vi "Write Autonomous.vi"() -> ()   [LabVIEW 2011]
uses:
  Shared/Autonomous Recording TypeDef.ctl
panel:
  in  "Autonomous Array":T1[](array[typedef])=[{"Left Drive Encoder"=0.0, "Right Drive Encoder"=0.0, "Shooter Mode"=enum."Off", "Set RPM"=0.0, "Set Motor Speed"=0.0, "Horn"=FALSE, "Shift Low"=FALSE, "Shift High"=FALSE, "Fire"=FALSE, "Reset Encoders"=FALSE}, {"Left Drive Encoder"=0.0, "Right Drive Encoder"=0.0, "Shooter Mode"=enum."Off", "Set RPM"=0.0, "Set Motor Speed"=0.0, "Horn"=FALSE, "Shift Low"=FALSE, "Shift High"=FALSE, "Fire"=FALSE, "Reset Encoders"=FALSE}, {"Left Drive Encoder"=0.0, "Right Drive Encoder"=0.0, "Shooter Mode"=enum."Off", "Set RPM"=0.0, "Set Motor Speed"=0.0, "Horn"=FALSE, "Shift Low"=FALSE, "Shift High"=FALSE, "Fire"=FALSE, "Reset Encoders"=FALSE}, {"Left Drive Encoder"=0.0, "Right Drive Encoder"=0.0, "Shooter Mode"=enum."Off", "Set RPM"=0.0, "Set Motor Speed"=0.0, "Horn"=FALSE, "Shift Low"=FALSE, "Shift High"=FALSE, "Fire"=FALSE, "Reset Encoders"=FALSE}, {"Left Drive Encoder"=0.0, "Right Drive Encoder"=0.0, "Shooter Mode"=enum."Off", "Set RPM"=0.0, "Set Motor Speed"=0.0, "Horn"=FALSE, "Shift Low"=FALSE, "Shift High"=FALSE, "Fire"=FALSE, "Reset Encoders"=FALSE}, {"Left Drive Encoder"=0.0, "Right Drive Encoder"=0.0, "Shooter Mode"=enum."Off", "Set RPM"=0.0, "Set Motor Speed"=0.0, "Horn"=FALSE, "Shift Low"=FALSE, "Shift High"=FALSE, "Fire"=FALSE, "Reset Encoders"=FALSE}, {"Left Drive Encoder"=0.0, "Right Drive Encoder"=0.0, "Shooter Mode"=enum."Off", "Set RPM"=0.0, "Set Motor Speed"=0.0, "Horn"=FALSE, "Shift Low"=FALSE, "Shift High"=FALSE, "Fire"=FALSE, "Reset Encoders"=FALSE}, {"Left Drive Encoder"=0.0, "Right Drive Encoder"=0.0, "Shooter Mode"=enum."Off", "Set RPM"=0.0, "Set Motor Speed"=0.0, "Horn"=FALSE, "Shift Low"=FALSE, "Shift High"=FALSE, "Fire"=FALSE, "Reset Encoders"=FALSE}, {"Left Drive Encoder"=0.0, "Right Drive Encoder"=0.0, "Shooter Mode"=enum."Off", "Set RPM"=0.0, "Set Motor Speed"=0.0, "Horn"=FALSE, "Shift Low"=FALSE, "Shift High"=FALSE, "Fire"=FALSE, "Reset Encoders"=FALSE}, {"Left Drive Encoder"=0.0, "Right Drive Encoder"=0.0, "Shooter Mode"=enum."Off", "Set RPM"=0.0, "Set Motor Speed"=0.0, "Horn"=FALSE, "Shift Low"=FALSE, "Shift High"=FALSE, "Fire"=FALSE, "Reset Encoders"=FALSE}, {"Left Drive Encoder"=0.0, "Right Drive Encoder"=0.0, "Shooter Mode"=enum."Off", "Set RPM"=0.0, "Set Motor Speed"=0.0, "Horn"=FALSE, "Shift Low"=FALSE, "Shift High"=FALSE, "Fire"=FALSE, "Reset Encoders"=FALSE}, {"Left Drive Encoder"=0.0, "Right Drive Encoder"=0.0, "Shooter Mode"=enum."Off", "Set RPM"=0.0, "Set Motor Speed"=0.0, "Horn"=FALSE, "Shift Low"=FALSE, "Shift High"=FALSE, "Fire"=FALSE, "Reset Encoders"=FALSE}, {"Left Drive Encoder"=0.0, "Right Drive Encoder"=0.0, "Shooter Mode"=enum."Off", "Set RPM"=0.0, "Set Motor Speed"=0.0, "Horn"=FALSE, "Shift Low"=FALSE, "Shift High"=FALSE, "Fire"=FALSE, "Reset Encoders"=FALSE}, {"Left Drive Encoder"=0.0, "Right Drive Encoder"=0.0, "Shooter Mode"=enum."Off", "Set RPM"=0.0, "Set Motor Speed"=0.0, "Horn"=FALSE, "Shift Low"=FALSE, "Shift High"=FALSE, "Fire"=FALSE, "Reset Encoders"=FALSE}, {"Left Drive Encoder"=0.0, "Right Drive Encoder"=0.0, "Shooter Mode"=enum."Off", "Set RPM"=0.0, "Set Motor Speed"=0.0, "Horn"=FALSE, "Shift Low"=FALSE, "Shift High"=FALSE, "Fire"=FALSE, "Reset Encoders"=FALSE}, {"Left Drive Encoder"=0.0, "Right Drive Encoder"=0.0, "Shooter Mode"=enum."Off", "Set RPM"=0.0, "Set Motor Speed"=0.0, "Horn"=FALSE, "Shift Low"=FALSE, "Shift High"=FALSE, "Fire"=FALSE, "Reset Encoders"=FALSE}, {"Left Drive Encoder"=0.0, "Right Drive Encoder"=0.0, "Shooter Mode"=enum."Off", "Set RPM"=0.0, "Set Motor Speed"=0.0, "Horn"=FALSE, "Shift Low"=FALSE, "Shift High"=FALSE, "Fire"=FALSE, "Reset Encoders"=FALSE}, {"Left Drive Encoder"=0.0, "Right Drive Encoder"=0.0, "Shooter Mode"=enum."Off", "Set RPM"=0.0, "Set Motor Speed"=0.0, "Horn"=FALSE, "Shift Low"=FALSE, "Shift High"=FALSE, "Fire"=FALSE, "Reset Encoders"=FALSE}, {"Left Drive Encoder"=0.0, "Right Drive Encoder"=0.0, "Shooter Mode"=enum."Off", "Set RPM"=0.0, "Set Motor Speed"=0.0, "Horn"=FALSE, "Shift Low"=FALSE, "Shift High"=FALSE, "Fire"=FALSE, "Reset Encoders"=FALSE}, {"Left Drive Encoder"=0.0, "Right Drive Encoder"=0.0, "Shooter Mode"=enum."Off", "Set RPM"=0.0, "Set Motor Speed"=0.0, "Horn"=FALSE, "Shift Low"=FALSE, "Shift High"=FALSE, "Fire"=FALSE, "Reset Encoders"=FALSE}, {"Left Drive Encoder"=0.0, "Right Drive Encoder"=0.0, "Shooter Mode"=enum."Off", "Set RPM"=0.0, "Set Motor Speed"=0.0, "Horn"=FALSE, "Shift Low"=FALSE, "Shift High"=FALSE, "Fire"=FALSE, "Reset Encoders"=FALSE}, {"Left Drive Encoder"=0.0, "Right Drive Encoder"=0.0, "Shooter Mode"=enum."Off", "Set RPM"=0.0, "Set Motor Speed"=0.0, "Horn"=FALSE, "Shift Low"=FALSE, "Shift High"=FALSE, "Fire"=FALSE, "Reset Encoders"=FALSE}, {"Left Drive Encoder"=0.0, "Right Drive Encoder"=0.0, "Shooter Mode"=enum."Off", "Set RPM"=0.0, "Set Motor Speed"=0.0, "Horn"=FALSE, "Shift Low"=FALSE, "Shift High"=FALSE, "Fire"=FALSE, "Reset Encoders"=FALSE}, {"Left Drive Encoder"=0.0, "Right Drive Encoder"=0.0, "Shooter Mode"=enum."Off", "Set RPM"=0.0, "Set Motor Speed"=0.0, "Horn"=FALSE, "Shift Low"=FALSE, "Shift High"=FALSE, "Fire"=FALSE, "Reset Encoders"=FALSE}, {"Left Drive Encoder"=0.0, "Right Drive Encoder"=0.0, "Shooter Mode"=enum."Off", "Set RPM"=0.0, "Set Motor Speed"=0.0, "Horn"=FALSE, "Shift Low"=FALSE, "Shift High"=FALSE, "Fire"=FALSE, "Reset Encoders"=FALSE}, {"Left Drive Encoder"=0.0, "Right Drive Encoder"=0.0, "Shooter Mode"=enum."Off", "Set RPM"=0.0, "Set Motor Speed"=0.0, "Horn"=FALSE, "Shift Low"=FALSE, "Shift High"=FALSE, "Fire"=FALSE, "Reset Encoders"=FALSE}, {"Left Drive Encoder"=0.0, "Right Drive Encoder"=0.0, "Shooter Mode"=enum."Off", "Set RPM"=0.0, "Set Motor Speed"=0.0, "Horn"=FALSE, "Shift Low"=FALSE, "Shift High"=FALSE, "Fire"=FALSE, "Reset Encoders"=FALSE}, {"Left Drive Encoder"=0.0, "Right Drive Encoder"=0.0, "Shooter Mode"=enum."Off", "Set RPM"=0.0, "Set Motor Speed"=0.0, "Horn"=FALSE, "Shift Low"=FALSE, "Shift High"=FALSE, "Fire"=FALSE, "Reset Encoders"=FALSE}, {"Left Drive Encoder"=0.0, "Right Drive Encoder"=0.0, "Shooter Mode"=enum."Off", "Set RPM"=0.0, "Set Motor Speed"=0.0, "Horn"=FALSE, "Shift Low"=FALSE, "Shift High"=FALSE, "Fire"=FALSE, "Reset Encoders"=FALSE}, {"Left Drive Encoder"=0.0, "Right Drive Encoder"=0.0, "Shooter Mode"=enum."Off", "Set RPM"=0.0, "Set Motor Speed"=0.0, "Horn"=FALSE, "Shift Low"=FALSE, "Shift High"=FALSE, "Fire"=FALSE, "Reset Encoders"=FALSE}, {"Left Drive Encoder"=0.0, "Right Drive Encoder"=0.0, "Shooter Mode"=enum."Off", "Set RPM"=0.0, "Set Motor Speed"=0.0, "Horn"=FALSE, "Shift Low"=FALSE, "Shift High"=FALSE, "Fire"=FALSE, "Reset Encoders"=FALSE}, {"Left Drive Encoder"=0.0, "Right Drive Encoder"=0.0, "Shooter Mode"=enum."Off", "Set RPM"=0.0, "Set Motor Speed"=0.0, "Horn"=FALSE, "Shift Low"=FALSE, "Shift High"=FALSE, "Fire"=FALSE, "Reset Encoders"=FALSE}, {"Left Drive Encoder"=0.0, "Right Drive Encoder"=0.0, "Shooter Mode"=enum."Off", "Set RPM"=0.0, "Set Motor Speed"=0.0, "Horn"=FALSE, "Shift Low"=FALSE, "Shift High"=FALSE, "Fire"=FALSE, "Reset Encoders"=FALSE}, {"Left Drive Encoder"=0.0, "Right Drive Encoder"=0.0, "Shooter Mode"=enum."Off", "Set RPM"=0.0, "Set Motor Speed"=0.0, "Horn"=FALSE, "Shift Low"=FALSE, "Shift High"=FALSE, "Fire"=FALSE, "Reset Encoders"=FALSE}, {"Left Drive Encoder"=0.0, "Right Drive Encoder"=0.0, "Shooter Mode"=enum."Off", "Set RPM"=0.0, "Set Motor Speed"=0.0, "Horn"=FALSE, "Shift Low"=FALSE, "Shift High"=FALSE, "Fire"=FALSE, "Reset Encoders"=FALSE}, {"Left Drive Encoder"=-1.7999999999999998, "Right Drive Encoder"=-1.7999999999999998, "Shooter Mode"=enum."Off", "Set RPM"=0.0, "Set Motor Speed"=0.0, "Horn"=FALSE, "Shift Low"=FALSE, "Shift High"=FALSE, "Fire"=FALSE, "Reset Encoders"=FALSE}, {"Left Drive Encoder"=-8.64, "Right Drive Encoder"=-6.12, "Shooter Mode"=enum."Off", "Set RPM"=0.0, "Set Motor Speed"=0.0, "Horn"=FALSE, "Shift Low"=FALSE, "Shift High"=FALSE, "Fire"=FALSE, "Reset Encoders"=FALSE}, {"Left Drive Encoder"=-14.399999999999999, "Right Drive Encoder"=-13.68, "Shooter Mode"=enum."Off", "Set RPM"=0.0, "Set Motor Speed"=0.0, "Horn"=FALSE, "Shift Low"=FALSE, "Shift High"=FALSE, "Fire"=FALSE, "Reset Encoders"=FALSE}, {"Left Drive Encoder"=-24.119999999999997, "Right Drive Encoder"=-27.36, "Shooter Mode"=enum."Off", "Set RPM"=0.0, "Set Motor Speed"=0.0, "Horn"=FALSE, "Shift Low"=FALSE, "Shift High"=FALSE, "Fire"=FALSE, "Reset Encoders"=FALSE}, {"Left Drive Encoder"=-36.36, "Right Drive Encoder"=0.0, "Shooter Mode"=enum."Off", "Set RPM"=0.0, "Set Motor Speed"=0.0, "Horn"=FALSE, "Shift Low"=FALSE, "Shift High"=FALSE, "Fire"=FALSE, "Reset Encoders"=FALSE}]
  in  "Path":path
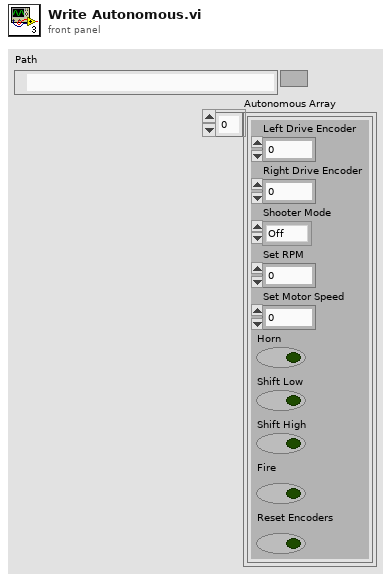
[diagram p1: front panel]
types:
  T1 = typedef "Autonomous Recording TypeDef.ctl" = cluster{"Left Drive Encoder":dbl, "Right Drive Encoder":dbl, "Shooter Mode":enum16{"Off", "Open Loop Control", "Closed Loop Control", "Top Spin"}, "Set RPM":dbl, "Set Motor Speed":dbl, "Horn":bool, "Shift Low":bool, "Shift High":bool, "Fire":bool, "Reset Encoders":bool}
  T2 = enum16{"open", "replace", "create", "open or create", "replace or create", "replace or create with confirmation"}
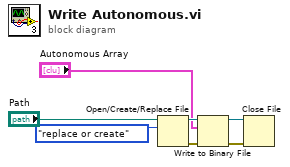
[diagram p0: block diagram]
diagram:
  n1 = Open/Create/Replace File(file path (use dialog)="Path", operation (0:open)=T2."replace or create") -> (refnum out=w6:refnum<file>, error out=w7:errorcluster)  [unwired: 4 in, 1 out]
  n2 = Write to Binary File(file (use dialog)=w6, data="Autonomous Array", error in=w7) -> (refnum out=w5:refnum<file>, error out=w4:errorcluster)  [unwired: 3 in, 1 out]
  n3 = Close File(refnum=w5, error in=w4) -> ()  [unwired: 2 out]
